vi "Main.vi"(11 "Module Admin":refnum<class "Delacor_lib_QMH_Module Admin.lvclass">) -> ()   [LabVIEW 2021, in "DAQ.lvlib"]
doc: "This template is based off of the Queued Message Handler design pattern and the Queued Message Handler project template that ships with LabVIEW.\n\nThe main difference is that the queue is private to this module and communication between modules is performed via Broadcast and Request events.\n\nRequest events are wrapped in public API methods and are handled in the Event Handling Loop (EHL) of this VI. Any module can register for Broadcast events sent by this module. The EHL generates messages based on user interface actions.\n\nThe Message Handling Loop (MHL) processes messages generated by the EHL, or by other messages. The messages are string values, so new messages can be added easily to the Message Cases case structure in the MHL. Each message cluster can also provide an optional value for Message Data, which is a variant that can be converted to whatever message-specific data is required.\n_____\nBased on Delacor QMH Project Template 5.0.0.82.\n\n<b>Note:</b> This VI was modified by the <b>Validate DQMH Module</b> tool to add a 'Panel Hidden' status updated broadcast to the Panel Close? event when External Launch = TRUE.\n\n<b>Note:</b> This VI was modified by the <b>Validate DQMH Module</b> tool to add a call to the Error Reported VI at the end of the 'Exit' MHL frame.\n\n<b>Note:</b> This VI was modified by the <b>Validate DQMH Module</b> tool to wrap the FP.Open method in the module close code with a Conditional Disable Structure so it does not execute when the Main VI is running as a built EXE."
uses:
  DAQ.lvlib
  <vilib>/Delacor/Delacor QMH/Libraries/Module Admin_class/Delacor_lib_QMH_Module Admin.lvclass
  Module Data--cluster.ctl
  <vilib>/Delacor/Delacor QMH/Libraries/Message Queue_class/Delacor_lib_QMH_Message Queue.lvclass/Delacor_lib_QMH_Message Queue.ctl
  Stop Argument--cluster.ctl
  <vilib>/Delacor/Delacor QMH/Libraries/Module Admin_class/Delacor_lib_QMH_Module Admin.lvclass/Delacor_lib_QMH_Module Admin.ctl
  Simulation Argument--cluster.ctl
  Set Output Argument--cluster.ctl
  td_cc_outputs.ctl
  Load in SubPane Argument--cluster.ctl
  UnLoad SubPane Argument--cluster.ctl
  <vilib>/Utility/miscctls.llb/LVPointTypeDef.ctl
  <vilib>/Delacor/Delacor QMH/Libraries/Message Queue_class/Delacor_lib_QMH_Enqueue Message (Single).vi
  <vilib>/Delacor/Delacor QMH/Libraries/Module Admin_class/Delacor_lib_QMH_Get External Launch.vi
  <vilib>/Utility/error.llb/Error Cluster From Error Code.vi
  <vilib>/ErrorRing/Error Ring.xnode
  <vilib>/Delacor/Delacor QMH/Libraries/Message Queue_class/Delacor_lib_QMH_Message Queue.lvclass
  Model/Model.lvlib
  <vilib>/DQMH Consortium/Lumos API/Libraries/SDV API/SDV API.lvlib
panel:
  out "Subpanel Ref":refnum<vi>
  in  "Sim":bool
  in  "DI3":bool
  in  "DI2":bool
  in  "DI1":bool
  in  "DI0":bool
  in  "DO3":bool
  in  "DO2":bool
  in  "DO1":bool
  in  "DO0":bool
  out "ModuleName":string
  out "Sim?":bool
  in  "ExitMod":bool
  in  "Simulate MHL Error":bool
  in  "Simulate EHL Error":bool
  out "error out":errorcluster
  out "Status":string
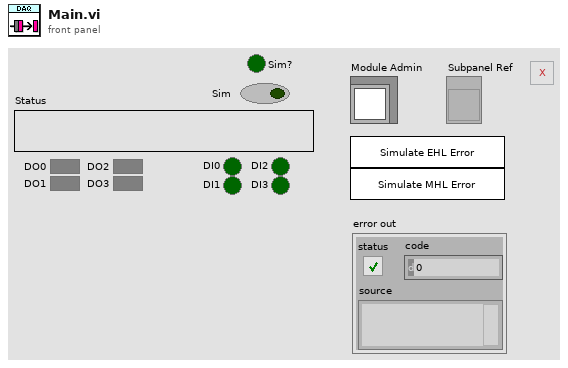
[diagram p1: front panel]
types:
  T1 = typedef "DAQ.lvlib/Request Events--cluster.ctl" = cluster{"Stop Module":refnum<user-event>, "Show Panel":refnum<user-event>, "Hide Panel":refnum<user-event>, "Get Module Execution Status":refnum<user-event>, "Show Diagram":refnum<user-event>, "Simulation":refnum<user-event>, "Set Output":refnum<user-event>, "Load in SubPane":refnum<user-event>, "UnLoad SubPane":refnum<user-event>}
  T2 = typedef "DAQ.lvlib/Module Data--cluster.ctl" = cluster{"Status":string, "Sim":bool}
  T3 = enum32{"invalid lock state", "Not Locked", "Locked (No Password)", "Password-protected"}
  T4 = typedef "DAQ.lvlib/Stop Argument--cluster.ctl" = cluster{"Origin":string, "Exit via Stop Module Req?":bool, "Wait for Module to stop?":bool}
  T5 = typedef "DAQ.lvlib/Simulation Argument--cluster.ctl" = cluster{"Sim?":bool}
  T6 = typedef "DAQ.lvlib/Set Output Argument--cluster.ctl" = cluster{"Outputs":T7}
  T7 = typedef "DAQ.lvlib/td_cc_outputs.ctl" = cluster{"DO00":bool, "DO01":bool, "DO02":bool, "DO03":bool, "DO04":bool}
  T8 = typedef "DAQ.lvlib/Load in SubPane Argument--cluster.ctl" = cluster{"Subpanel Ref":refnum<vi>}
  T9 = typedef "DAQ.lvlib/UnLoad SubPane Argument--cluster.ctl" = cluster{"Subpanel Ref":refnum<vi>}
  T10 = typedef "LVPointTypeDef.ctl" = cluster{"Horizontal":i16, "Vertical":i16}
  T11 = enum32{"Invalid", "Standard", "Closed", "Hidden", "Minimized", "Maximized"}
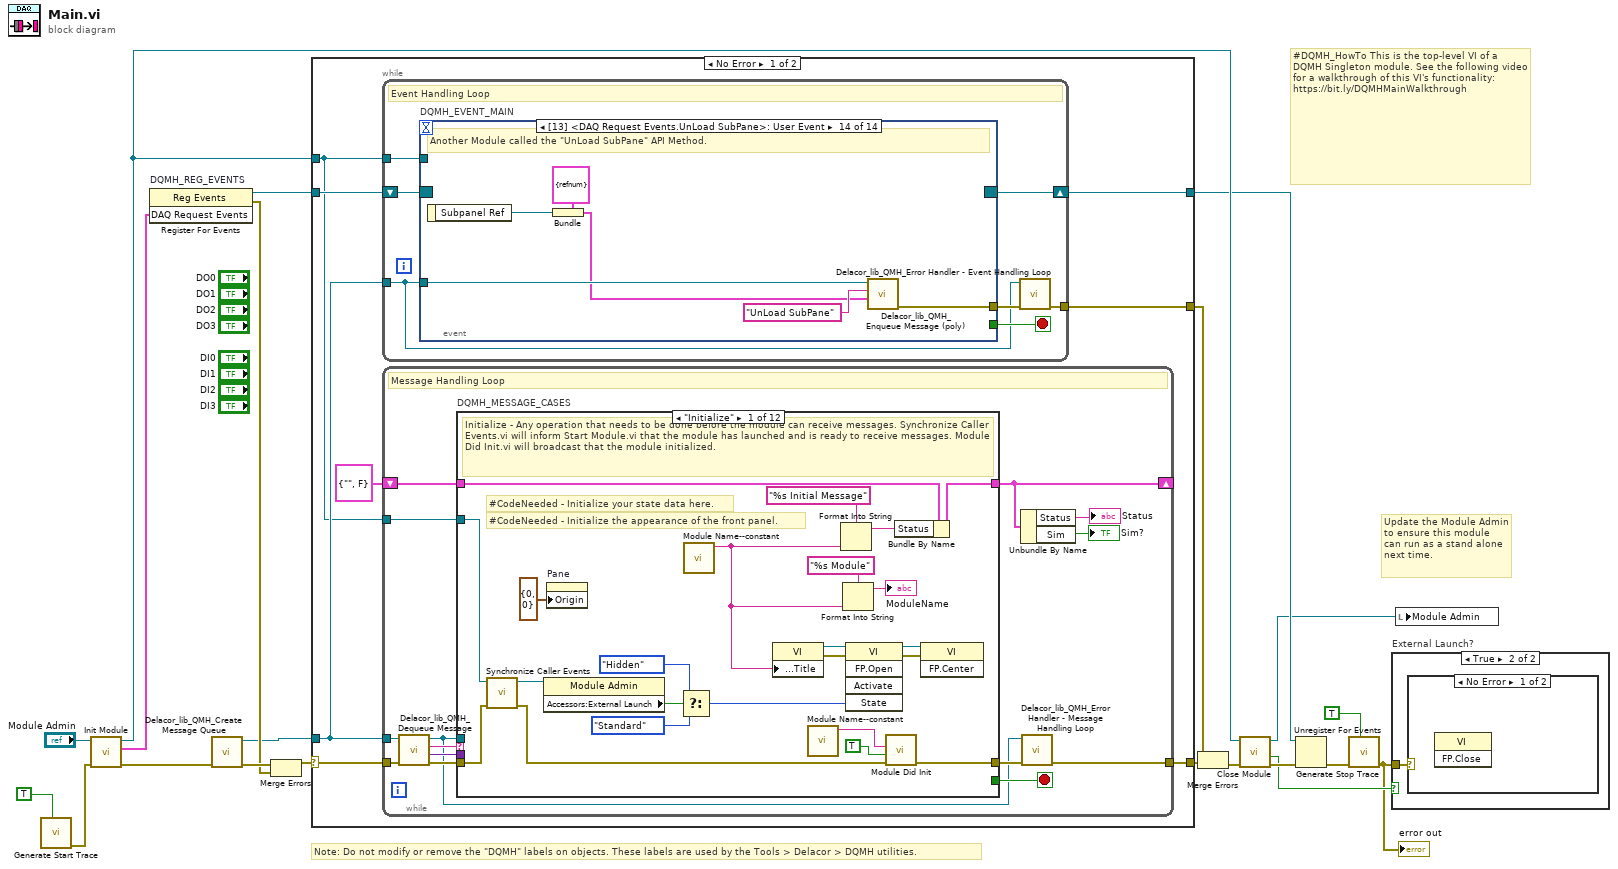
[diagram p0: block diagram]
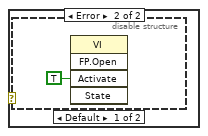
[diagram p3: hidden frame]
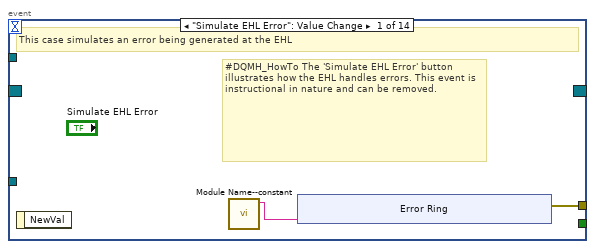
[diagram p5: hidden frame]
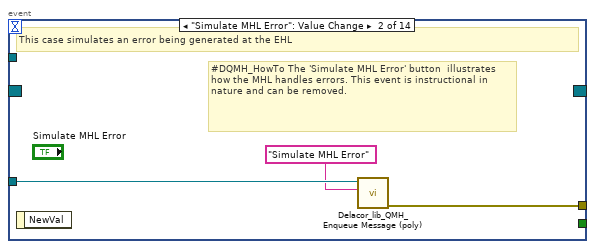
[diagram p6: hidden frame]
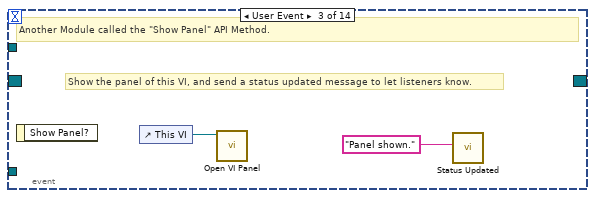
[diagram p7: hidden frame]
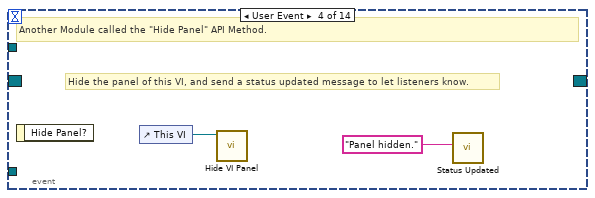
[diagram p8: hidden frame]
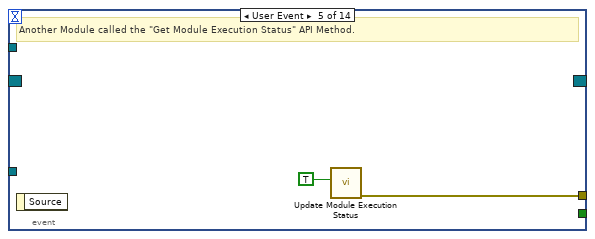
[diagram p9: hidden frame]
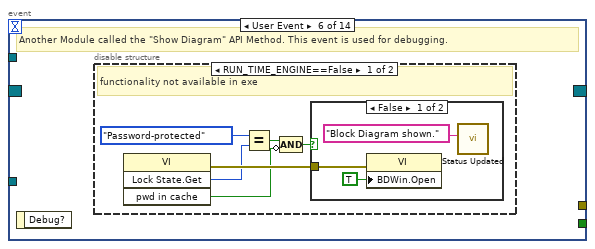
[diagram p10: hidden frame]
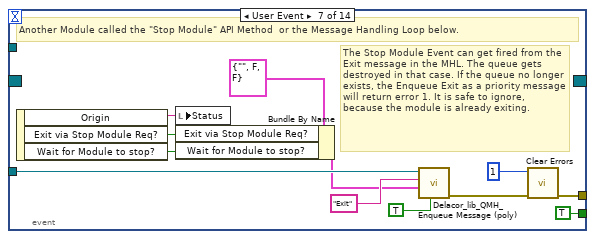
[diagram p13: hidden frame]
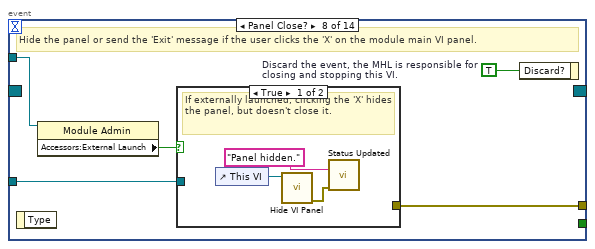
[diagram p14: hidden frame]
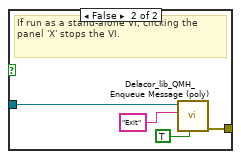
[diagram p15: hidden frame]
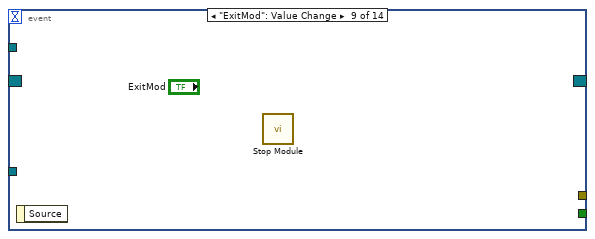
[diagram p16: hidden frame]
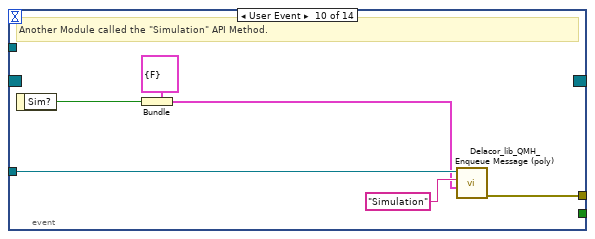
[diagram p17: hidden frame]
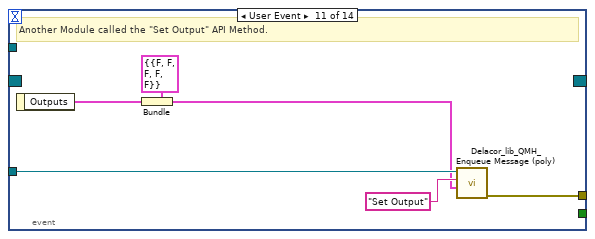
[diagram p18: hidden frame]
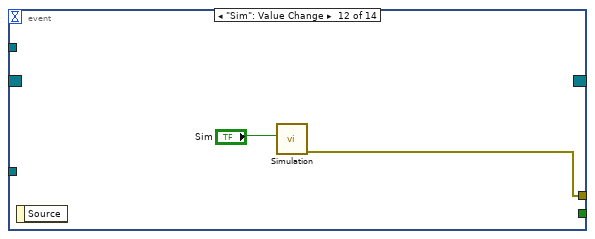
[diagram p19: hidden frame]
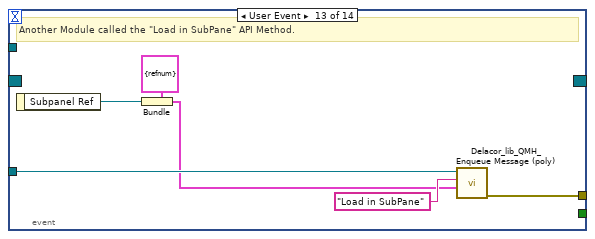
[diagram p20: hidden frame]
diagram:
  # "#DQMH_HowTo This is the top-level VI of a DQMH Singleton module. See the following video for a walkthrough of this VI's functionality: https://bit.ly/DQMHMainWalkthrough"
  # "Note: Do not modify or remove the \"DQMH\" labels on objects. These labels are used by the Tools > Delacor > DQMH utilities."
  # "Update the Module Admin to ensure this module can run as a stand alone next time."
  n1 = call <vilib>:"Generate Start Trace.vi"("Reply (F)"=TRUE) -> ("error out"=w4:errorcluster)  [unwired: 10 in]
  n2 = call "Init Module.vi"("error in (no error)"=w4, "Singleton Module Admin in"="Module Admin") -> ("error out"=w20:errorcluster, "DAQ Request Events"=w9:T1, "Singleton Module Admin out"=w12:refnum<class "Delacor_lib_QMH_Module Admin.lvclass">)  [unwired: 7 in]
  n3 = register-events "DQMH_REG_EVENTS"(w9) -> (reference out=w10:refnum<event-registration>, error out=w13:errorcluster)  [unwired: 2 in]
  n4 = call <vilib>:"Delacor_lib_QMH_Create Message Queue.vi"("error in"=w20) -> ("error out"=w15:errorcluster, "Message Queue"=w8:refnum<class "Delacor_lib_QMH_Message Queue.lvclass">)  [unwired: 9 in]
  n5 = Merge Errors(w15, w13) -> (w14:errorcluster)
  n6 = case shown="No Error" w14 {
    selector: w14 -> [w27 w254]
    tunnel: [w29 w253] -> w21
    tunnel: [w26 w259] -> w11
    tunnel: w10 -> [w24 w259]
    tunnel: w8 -> [w23 w252]
    tunnel: [w28 _] -> w18
    tunnel: w12 -> [w22 w255]
    frame No Error {
      n7 = while {
        tunnel: w23 -> [w30]
        shift-right: [w33] -> w26
        shift-left: w24 -> [w34]
        tunnel: [w35] -> w28
        tunnel: w22 -> [w31]
        stop <- w32 stop-if-true
        # "Event Handling Loop"
        n8 = event "DQMH_EVENT_MAIN" shown="[13] <DAQ Request Events.UnLoad SubPane>: User Event" {
          selector: w34 -> [_ _ _ _ _ _ _ _ _ _ _ _ _ _]
          dyn-events: [_ _ _ _ _ _ _ _ _ _ _ _ _ _] -> w33
          timeout: _ -> [_ _ _ _ _ _ _ _ _ _ _ _ _ _]
          tunnel: [_ _ _ _ _ _ TRUE ("Discard?") _ _ _ _ _ _ _] -> w32
          tunnel: w30 -> [_ w47 _ _ _ _ w71 w78 _ w93 w99 _ w107 w113]
          tunnel: [w38 w48 _ _ w54 _ w74 w80 _ w88 w94 w101 w102 w108] -> w36
          tunnel: w31 -> [_ _ _ _ _ _ _ w77 _ _ _ _ _ _]
          event "Simulate EHL Error": Value Change {
            # "#DQMH_HowTo The 'Simulate EHL Error' button  illustrates how the EHL handles errors. This event is instructional in nature and can be removed."
            # "This case simulates an error being generated at the EHL"
            n9 = event-data() -> ()  [unwired: 1 in, 1 out]
            n10 = call "Module Name--constant.vi"() -> ("Module Name"=w37:string)  [unwired: 11 in]
            n11 = xnode ("Error Ring")("parameter 0"=w37) -> ("error out"=w38:errorcluster)
          }
          event "Simulate MHL Error": Value Change {
            # "#DQMH_HowTo The 'Simulate MHL Error' button  illustrates how the MHL handles errors. This event is instructional in nature and can be removed."
            # "This case simulates an error being generated at the EHL"
            n12 = event-data() -> ()  [unwired: 1 in, 1 out]
            n13 = call-poly <vilib>:"Delacor_lib_QMH_Enqueue Message (poly).vi"("Message"="Simulate MHL Error", "Message Queue in"=w47) -> ("error out"=w48:errorcluster)  [unwired: 8 in, 1 out]
          }
          event User Event {
            # "Show the panel of this VI, and send a status updated message to let listeners know."
            # "Another Module called the \"Show Panel\" API Method."
            n14 = event-data() -> ()  [unwired: 1 in, 1 out]
            n15 = control-ref of="This VI"() -> (w50:refnum<vi>)
            n16 = call "Open VI Panel.vi"("VI"=w50) -> ()  [unwired: 10 in, 1 out]
            n17 = call "Status Updated.vi"("Status"="Panel shown." ("format string")) -> ()  [unwired: 10 in, 1 out]
          }
          event User Event {
            # "Hide the panel of this VI, and send a status updated message to let listeners know."
            # "Another Module called the \"Hide Panel\" API Method."
            n18 = event-data() -> ()  [unwired: 1 in, 1 out]
            n19 = control-ref of="This VI"() -> (w52:refnum<vi>)
            n20 = call "Hide VI Panel.vi"("VI"=w52) -> ()  [unwired: 10 in, 1 out]
            n21 = call "Status Updated.vi"("Status"="Panel hidden." ("format string")) -> ()  [unwired: 10 in, 1 out]
          }
          event User Event {
            # "Another Module called the \"Get Module Execution Status\" API Method."
            n22 = event-data() -> ()  [unwired: 1 in, 1 out]
            n23 = call "Update Module Execution Status.vi"("Running?"=TRUE) -> ("error out"=w54:errorcluster)  [unwired: 10 in]
          }
          event User Event {
            # "Another Module called the \"Show Diagram\" API Method. This event is used for debugging."
            n24 = event-data() -> ()  [unwired: 1 in, 1 out]
            n25 = disable-structure "Conditional Disable Structure" shown="RUN_TIME_ENGINE==False" {
              frame condition #0 (active) {
                # "functionality not available in exe"
                n26 = invoke on="Invoke Node" class="VI" method="Lock State.Get"() -> (error out=w60:errorcluster, "Get Lock State"=w59:T3, "pwd in cache"=w56:bool)  [unwired: 4 in, 1 out]
                n27 = Equal?(x=T3."Password-protected", y=w59) -> (x = y?=w57:bool)
                n28 = Compound Arithmetic op=AND(w57, invert w56) -> (w55:bool)
                n29 = case shown="False" w55 {
                  tunnel: w60 -> [w63 _]
                  frame False {
                    n30 = property on="Property Node" class="VI"(error in=w63, "BDWin.Open"=TRUE ("Block Diagram Window:Open")) -> ()  [unwired: 1 in, 2 out]
                    n31 = call "Status Updated.vi"("Status"="Block Diagram shown." ("format string")) -> ()  [unwired: 10 in, 1 out]
                  }
                  frame True {
                    # "Password-protected VI, and the password is not in the cache. Do not show the diagram."
                  }
                }
              }
              frame condition #1 {
              }
            }
          }
          event User Event {
            # "The Stop Module Event can get fired from the Exit message in the MHL. The queue gets destroyed in that case. If the queue no longer exists, the Enqueue Exit as a priority message will return error 1. It is safe to ignore, because the module is already exiting."
            # "Another Module called the \"Stop Module\" API Method  or the Message Handling Loop below."
            n32 = event-data() -> ("Origin"=w70:string, "Exit via Stop Module Req?"=w66:bool, "Wait for Module to stop?"=w65:bool)  [unwired: 1 in]
            n33 = local write "Status"(w70) -> ()
            n34 = Bundle By Name(cluster=T4 {"Origin"="", "Exit via Stop Module Req?"=FALSE, "Wait for Module to stop?"=FALSE} ("Stop Argument"), "Exit via Stop Module Req?"=w66, "Wait for Module to stop?"=w65) -> (w64:T4)
            n35 = call-poly <vilib>:"Delacor_lib_QMH_Enqueue Message (poly).vi"("Priority Message? (F)"=TRUE, "Message Data"=w64, "Message"="Exit", "Message Queue in"=w71) -> ("error out"=w75:errorcluster)  [unwired: 6 in, 1 out]
            n36 = call <vilib>:"Clear Errors.vi"("error in (no error)"=w75, "specific error code to clear (0: all)"=1) -> ("error out"=w74:errorcluster)  [unwired: 4 in, 1 out]
          }
          event Panel Close? {
            w79 = TRUE  # Discard the event, the MHL is responsible for closing and stopping this VI.
            # "Hide the panel or send the 'Exit' message if the user clicks the 'X' on the module main VI panel."
            n37 = event-data() -> ()  [unwired: 1 in, 1 out]
            n38 = property on="Property Node" class="Module Admin"(reference=w77) -> ("Accessors:External Launch"=w76:bool)  [unwired: 1 in, 2 out]
            n39 = case shown="True" w76 {
              tunnel: w78 -> [_ w86]
              tunnel: [_ w87] -> w80
              frame True {
                # "If externally launched, clicking the 'X' hides the panel, but doesn't close it."
                n40 = control-ref of="This VI"() -> (w83:refnum<vi>)
                n41 = call "Hide VI Panel.vi"("VI"=w83) -> ("error out"=w81:errorcluster)  [unwired: 10 in]
                n42 = call "Status Updated.vi"("error in (no error)"=w81, "Status"="Panel hidden.") -> ()  [unwired: 9 in, 1 out]
              }
              frame False {
                # "If run as a stand-alone VI, clicking the panel 'X' stops the VI."
                n43 = call-poly <vilib>:"Delacor_lib_QMH_Enqueue Message (poly).vi"("Priority Message? (F)"=TRUE, "Message"="Exit", "Message Queue in"=w86) -> ("error out"=w87:errorcluster)  [unwired: 7 in, 1 out]
              }
            }
            n44 = event-data ("Event Filter Node")("Discard?"=w79) -> ()  [unwired: 1 in, 1 out]
          }
          event "ExitMod": Value Change {
            n45 = event-data() -> ()  [unwired: 1 in, 1 out]
            n46 = call "Stop Module.vi"() -> ()  [unwired: 11 in, 1 out]
          }
          event User Event {
            # "Another Module called the \"Simulation\" API Method."
            n47 = event-data() -> ("Sim?"=w89:bool)  [unwired: 1 in]
            n48 = Bundle(cluster=T5 {"Sim?"=FALSE} ("Simulation Argument"), "Sim?"=w89) -> (w90:T5)
            n49 = call-poly <vilib>:"Delacor_lib_QMH_Enqueue Message (poly).vi"("Message Data"=w90, "Message"="Simulation", "Message Queue in"=w93) -> ("error out"=w88:errorcluster)  [unwired: 7 in, 1 out]
          }
          event User Event {
            # "Another Module called the \"Set Output\" API Method."
            n50 = event-data() -> ("Outputs"=w95:T7)  [unwired: 1 in]
            n51 = Bundle(cluster=T6 {"Outputs"={"DO00"=FALSE, "DO01"=FALSE, "DO02"=FALSE, "DO03"=FALSE, "DO04"=FALSE}} ("Set Output Argument"), "Outputs"=w95) -> (w96:T6)
            n52 = call-poly <vilib>:"Delacor_lib_QMH_Enqueue Message (poly).vi"("Message Data"=w96, "Message"="Set Output", "Message Queue in"=w99) -> ("error out"=w94:errorcluster)  [unwired: 7 in, 1 out]
          }
          event "Sim": Value Change {
            n53 = event-data() -> ()  [unwired: 1 in, 1 out]
            n54 = call "Simulation.vi"("Sim?"="Sim") -> ("error out"=w101:errorcluster)  [unwired: 10 in]
          }
          event User Event {
            # "Another Module called the \"Load in SubPane\" API Method."
            n55 = event-data() -> ("Subpanel Ref"=w103:refnum<vi>)  [unwired: 1 in]
            n56 = Bundle(cluster=T8 {"Subpanel Ref"=refnum} ("Load in SubPane Argument"), "Subpanel Ref"=w103) -> (w104:T8)
            n57 = call-poly <vilib>:"Delacor_lib_QMH_Enqueue Message (poly).vi"("Message Data"=w104, "Message"="Load in SubPane", "Message Queue in"=w107) -> ("error out"=w102:errorcluster)  [unwired: 7 in, 1 out]
          }
          event User Event {
            # "Another Module called the \"UnLoad SubPane\" API Method."
            n58 = event-data() -> ("Subpanel Ref"=w109:refnum<vi>)  [unwired: 1 in]
            n59 = Bundle(cluster=T9 {"Subpanel Ref"=refnum} ("UnLoad SubPane Argument"), "Subpanel Ref"=w109) -> (w110:T9)
            n60 = call-poly <vilib>:"Delacor_lib_QMH_Enqueue Message (poly).vi"("Message Data"=w110, "Message"="UnLoad SubPane", "Message Queue in"=w113) -> ("error out"=w108:errorcluster)  [unwired: 7 in, 1 out]
          }
        }
        n61 = call-dynamic "Delacor_lib_QMH_Error Handler - Event Handling Loop.vi"("error in"=w36, "Message Queue in"=w30) -> ("dup error in"=w35:errorcluster)  [unwired: 8 in, 1 out]
      }
      n62 = while {
        tunnel: w23 -> [w119]
        shift-right: [w116] -> _
        shift-left: T2 {"Status"="", "Sim"=FALSE} ("Data Cluster") -> [w123]
        tunnel: w27 -> [w126]
        tunnel: [w124] -> w29
        tunnel: w22 -> [w117]
        stop <- w122 stop-if-true
        # "Message Handling Loop"
        n63 = call-dynamic "Delacor_lib_QMH_Dequeue Message.vi"("error in"=w126, "Message Queue in"=w119) -> ("error out"=w125:errorcluster, "Message Data"=w120:variant, "Message"=w121:string, "Message Queue out"=w118:refnum<class "Delacor_lib_QMH_Message Queue.lvclass">)  [unwired: 6 in]
        n64 = case "DQMH_MESSAGE_CASES" shown="\"Initialize\"" w121 {
          selector: w121 -> [_ _ w159 _ _ _ _ _ _ _ _ w239]
          tunnel: w118 -> [_ _ _ _ _ _ _ _ _ w207 w231 _]
          tunnel: w125 -> [w148 w152 w166 w172 w180 w187 w190 w192 w197 w214 w237 w241]
          tunnel: [w146 w152 w164 w170 w178 w185 w189 w192 w196 w210 w234 w242] -> w127
          tunnel: w123 -> [w139 w151 w165 w171 w179 w186 w188 w191 w194 w209 w230 w240]
          tunnel: [w138 w151 w160 w171 w179 w186 w188 w191 w194 w209 w230 w240] -> w116
          tunnel: [_ _ _ _ _ _ _ _ _ _ w229 _] -> w122
          tunnel: w120 -> [_ _ w163 w169 w177 w184 _ _ _ w208 w228 _]
          tunnel: w117 -> [w140 _ _ _ _ _ _ _ _ w206 w223 _]
          frame "Initialize" {
            # "#CodeNeeded - Initialize the appearance of the front panel."
            # "#CodeNeeded - Initialize your state data here."
            # "Initialize - Any operation that needs to be done before the module can receive messages. Synchronize Caller Events.vi will inform Start Module.vi that the module has launched and is ready to receive messages. Module Did Init.vi will broadcast that the module initialized."
            n65 = call "Synchronize Caller Events.vi"("error in (no error)"=w148, "Singleton Module Admin in"=w140) -> ("error out"=w147:errorcluster, "Singleton Module Admin out"=w135:refnum<class "Delacor_lib_QMH_Module Admin.lvclass">)  [unwired: 8 in]
            n66 = property on="Property Node" class="Module Admin"(reference=w135) -> ("Accessors:External Launch"=w144:bool)  [unwired: 1 in, 2 out]
            n67 = property on="Pane" class="Pane"("Origin"=T10 {"Horizontal"=0, "Vertical"=0}) -> ()  [unwired: 2 in, 2 out]
            n68 = Select(t=T11."Hidden" ("State"), s=w144, f=T11."Standard" ("State")) -> (s? t:f=w141:T11)
            n69 = call "Module Name--constant.vi"() -> ("Module Name"=w131:string)  [unwired: 11 in]
            n70 = property on="Property Node" class="VI"("Front Panel.Title"=w131) -> (reference out=w145:refnum<vi>, error out=w150:errorcluster)  [unwired: 2 in]
            n71 = call "Module Name--constant.vi"() -> ("Module Name"=w136:string)  [unwired: 11 in]
            n72 = Format Into String(format string="%s Initial Message" ("Initial Message"), w131) -> (resulting string=w133:string)  [unwired: 2 in, 1 out]
            n73 = Format Into String(format string="%s Module", w131) -> (resulting string=→"ModuleName":string)  [unwired: 2 in, 1 out]
            n74 = invoke on="Invoke Node" class="VI" method="FP.Open"(reference=w145, error in=w150, "State"=w141) -> (reference out=w128:refnum<vi>, error out=w149:errorcluster)  [unwired: 2 in, 3 out]
            n75 = call "Module Did Init.vi"("error in (no error)"=w147, "Initialized?"=TRUE, "Origin"=w136) -> ("error out"=w146:errorcluster)  [unwired: 8 in]
            n76 = Bundle By Name(cluster=w139, "Status"=w133) -> (w138:T2)
            n77 = invoke on="Invoke Node" class="VI" method="FP.Center"(reference=w128, error in=w149) -> ()  [unwired: 1 in, 3 out]
          }
          frame "--- Module Specific ---" {
            # "Separator -- The following cases handle messages specific to this Module."
          }
          frame "Simulation" {
            # "This will change Module into Simulation Mode"
            n78 = Variant To Data(error in=w166, type=T5 {"Sim?"=FALSE} ("Simulation Argument"), Variant=w163) -> (data=w161:T5, error out=w164:errorcluster)
            n79 = Unbundle By Name(w161) -> ("Sim?"=w158:bool)
            n80 = Select(t="True", s=w158, f="False") -> (s? t:f=w154:string)
            n81 = Format Into String(format string="%s: %s", w159, w154) -> (resulting string=w153:string)  [unwired: 2 in, 1 out]
            n82 = Bundle By Name(cluster=w165, "Status"=w153, "Sim"=w158) -> (w160:T2)
          }
          frame "Set Output" {
            # "#CodeNeeded\n1. Configure this Message Case for handling the \"Set Output\" message.\n2. Delete or edit this label when done."
            # "This will set outputs"
            n83 = Variant To Data(error in=w172, type=T6 {"Outputs"={"DO00"=FALSE, "DO01"=FALSE, "DO02"=FALSE, "DO03"=FALSE, "DO04"=FALSE}} ("Set Output Argument"), Variant=w169) -> (data=w167:T6, error out=w170:errorcluster)
            n84 = Unbundle By Name(w167) -> ()  [unwired: 1 out]
          }
          frame "Load in SubPane" {
            n85 = Variant To Data(error in=w180, type=T8 {"Subpanel Ref"=refnum} ("Load in SubPane Argument"), Variant=w177) -> (data=w175:T8, error out=w178:errorcluster)
            n86 = Unbundle By Name(w175) -> ("Subpanel Ref"=w173:refnum<vi>)
            "Subpanel Ref" <- w173
            n87 = control-ref of="This VI"() -> (w174:refnum<vi>)
            n88 = call "Insert SubPanl.vi"("VI Ref"=w174, "Subpanel Ref"=w173) -> ()  [unwired: 9 in, 1 out]
          }
          frame "UnLoad SubPane" {
            n89 = Variant To Data(error in=w187, type=T9 {"Subpanel Ref"=refnum} ("UnLoad SubPane Argument"), Variant=w184) -> (data=w182:T9, error out=w185:errorcluster)
            n90 = Unbundle By Name(w182) -> ("Subpanel Ref"=w181:refnum<vi>)
            n91 = call "Remove SubPanel.vi"("Subpanel Ref"=w181) -> ()  [unwired: 10 in, 1 out]
          }
          frame "---Copy This Frame---" {
            # "Duplicate this frame when creating new messages.  Change this comment in the duplicated frame to describe this message."
            n92 = Merge Errors(w190) -> (w189:errorcluster)
          }
          frame "--- Exit and Error Handling---" {
            # "Separator - The following cases handle errors and exit messages."
          }
          frame "Simulate MHL Error" {
            # "#DQMH_HowTo The 'Simulate MHL Error' button  illustrates how the MHL handles errors. This event is instructional in nature and can be removed."
            # "Simulate an error occurring at the MHL"
            n93 = call "Module Name--constant.vi"() -> ("Module Name"=w193:string)  [unwired: 11 in]
            n94 = xnode ("Error Ring")("parameter 0"=w193) -> ("error out"=w195:errorcluster)
            n95 = Merge Errors(w197, w195) -> (w196:errorcluster)
          }
          frame "Error" {
            # "#CodeRecommended - If you ever change the name of this \"Error\" message, you'll need to update the name in the Check Loop Error.vi as well."
            # "#CodeRecommended - If the module is running in standalone mode (External Launch = FALSE), this code will pop up an error dialog and call the 'Exit' message if an error occurs. Add more fine-grained error handling here."
            # "Error - Check the error message data and respond accordingly. This message is sent by the \"Error Handler\" VIs at the end of each loop in this application."
            n96 = property on="Property Node" class="Module Admin"(reference=w206) -> ("Accessors:External Launch"=w205:bool)  [unwired: 1 in, 2 out]
            n97 = Variant To Data(error in=w214, type=errorcluster {"status"=FALSE, "code"=0, "source"=""} ("error constant"), Variant=w208) -> (data=w215:errorcluster, error out=w212:errorcluster)
            n98 = call "Error Reported.vi"("Error"=w215) -> ()  [unwired: 10 in, 1 out]
            n99 = case shown="False" w205 {
              tunnel: [w220 _] -> w211
              tunnel: w207 -> [w218 _]
              tunnel: w215 -> [w219 _]
              frame False {
                # "If the module is running standalone, then pop up an error dialog and call the \"Exit\" message."
                n100 = call <vilib>:"Simple Error Handler.vi"("error in (no error)"=w219) -> ()  [unwired: 4 in, 5 out]
                n101 = call-poly <vilib>:"Delacor_lib_QMH_Enqueue Message (poly).vi"("Priority Message? (F)"=TRUE, "Message"="Exit", "Message Queue in"=w218) -> ("error out"=w220:errorcluster)  [unwired: 7 in, 1 out]
              }
              frame True {
                # "If the module was launched externally, calling the Error Reported broadcast VI is the only action performed by the \"Error\" message. The module's caller can then process the error appropriately."
              }
            }
            n102 = Merge Errors(w212, w211) -> (w210:errorcluster)
            n103 = local write "error out"(w210) -> ()
          }
          frame "Exit" {
            w227 = 91  # 91: not all Exit messages will have an argument
            w229 = TRUE  # Stop the VI
            # "Release the message queue reference"
            # "Exit - Exit the application."
            n104 = Variant To Data(error in=w237, type=T4 {"Origin"="", "Exit via Stop Module Req?"=FALSE, "Wait for Module to stop?"=FALSE} ("Stop Argument"), Variant=w228) -> (data=w225:T4, error out=w233:errorcluster)
            n105 = call <vilib>:"Clear Errors.vi"("error in (no error)"=w233, "specific error code to clear (0: all)"=w227) -> ("error out"=w236:errorcluster)  [unwired: 4 in, 1 out]
            n106 = local read "Subpanel Ref"() -> (w221:refnum<vi>)
            n107 = control-ref of="This VI"() -> (w224:refnum<vi>)
            n108 = call "Remove SubPanel.vi"("Subpanel Ref"=w221) -> ("error out"=w222:errorcluster)  [unwired: 10 in]
            n109 = call-dynamic "Delacor_lib_QMH_Release Message Queue.vi"("error in"=w236, "Message Queue"=w231) -> ("error out"=w235:errorcluster)  [unwired: 9 in]
            n110 = call "Handle Exit.vi"("error in (no error)"=w222, "Stop Argument"=w225, "Admin in"=w223, "VI reference"=w224) -> ("error out"=w232:errorcluster)  [unwired: 6 in, 1 out]
            n111 = Merge Errors(w235, w232) -> (w234:errorcluster)
            n112 = call "Error Reported.vi"("Error"=w234) -> ()  [unwired: 10 in, 1 out]
          }
          frame Default {
            # "'Default' case only runs if there is a message that isn't defined in any of the other cases.  Output a programming error."
            n113 = call "Module Name--constant.vi"() -> ("Module Name"=w238:string)  [unwired: 11 in]
            n114 = xnode ("Error Ring")("parameter 0"=w239, "parameter 1"=w238) -> ("error out"=w243:errorcluster)
            n115 = Merge Errors(w241, w243) -> (w242:errorcluster)
          }
        }
        n116 = Unbundle By Name(w116) -> ("Status"=→"Status":string, "Sim"=→"Sim?":bool)
        n117 = call-dynamic "Delacor_lib_QMH_Error Handler - Message Handling Loop.vi"("error in"=w127, "Message Queue in"=w118) -> ("dup error in"=w124:errorcluster)  [unwired: 8 in, 1 out]
      }
    }
    frame Error {
      # "Synchronize Caller Events.vi will inform Start Module.vi that the module has launched and will let the code calling Start Module.vi register for broadcasts and would permit the caller receive the broadcast that an error occurred at launch time."
      n118 = call-dynamic "Delacor_lib_QMH_Release Message Queue.vi"("error in"=w254, "Message Queue"=w252) -> ("error out"=w253:errorcluster)  [unwired: 9 in]
      n119 = call "Synchronize Caller Events.vi"("Singleton Module Admin in"=w255) -> ("error out"=w260:errorcluster)  [unwired: 9 in, 1 out]
      n120 = call "Module Name--constant.vi"() -> ("Module Name"=w258:string)  [unwired: 11 in]
      n121 = Format Into String(format string="An error occurred during initialization. %s is no longer running.", w258) -> (resulting string=w256:string)  [unwired: 2 in, 1 out]
      n122 = Merge Errors(w253, w260) -> (w261:errorcluster)
      n123 = call "Error Reported.vi"("Additional Information"=w256, "Error"=w261) -> ()  [unwired: 9 in, 1 out]
    }
  }
  n124 = Merge Errors(w18, w21) -> (w17:errorcluster)
  n125 = call "Close Module.vi"("error in (no error)"=w17, "Module Admin in"=w12) -> ("error out"=w19:errorcluster, "External Launch"=w5:bool, "Module Admin out"=w6:refnum<class "Delacor_lib_QMH_Module Admin.lvclass">)  [unwired: 7 in]
  n126 = Unregister For Events(event registration refnum=w11, error in=w19) -> (error out=w16:errorcluster)
  n127 = call <vilib>:"Generate Stop Trace.vi"("Reply (F)"=TRUE, "error in (no error)"=w16) -> ("error out"=w2:errorcluster)  [unwired: 9 in]
  "error out" <- w2
  n128 = case "External Launch?" shown="True" w5 {
    tunnel: w2 -> [_ w262]
    frame False {
    }
    frame True {
      n129 = case shown="No Error" w262 {
        frame No Error {
          n130 = invoke on="Invoke Node" class="VI" method="FP.Close"() -> ()  [unwired: 3 in, 3 out]
        }
        frame Error {
          n131 = disable-structure shown="Default" {
            frame condition #0 (active) {
              n132 = invoke class="VI" method="FP.Open"("Activate"=TRUE ("Activate?")) -> ()  [unwired: 4 in, 5 out]
            }
            frame condition #1 {
              # "Don't show panel on error if running inside a built EXE."
            }
          }
        }
      }
    }
  }
  n133 = local write "Module Admin"(w6) -> ()
